vi "Simple Serial.vi"() -> ()   [LabVIEW 2021]
doc: "This example performs a serial port write and a serial port read. The parameters set for the serial port must match the parameters of the connected instrument or device. The VISA Configure Serial Port VI sets the configuration parameters. The front panel displays the controls used to configure the basic parameters, such as baud rate, data bits, and parity. The VI passes the VISA resource name to other VIs that perform operations on that VISA resource. The VISA Write function sends a command to the serial device and the VISA Read function returns data based on the command. The VISA Close function then closes the reference to the serial device. It is important to close the reference; otherwise, further communication through that port might not be possible."
uses:
  <vilib>/Instr/_visa.llb/VISA Open Access Mode.ctl
  <vilib>/Instr/_visa.llb/VISA Configure Serial Port (Instr).vi
panel:
  in  "Command":string="CAB-2558\n"
  out "bytes read":u32
  in  "delay before read (ms)":u32=500
  out "Response":string
  in  "VISA resource name":refnum<visa-resource-name>="COM1"
  # "Overview: Demonstrates the use of the VISA functions to send a single command to a serial instrument and read a response.\nRequirements: NI-VISA Driver\nInstructions:\n1. Ensure the resource specified by the VISA resource name is a valid serial device.\n2. Run the VI.\n3. If your instrument recognizes the \"*IDN?\" command, it should return a Response."
  # "Note: For an example of how to perform continuous serial communication in a loop, open the Continuous Serial Write and Read.vi in the same folder as this example."
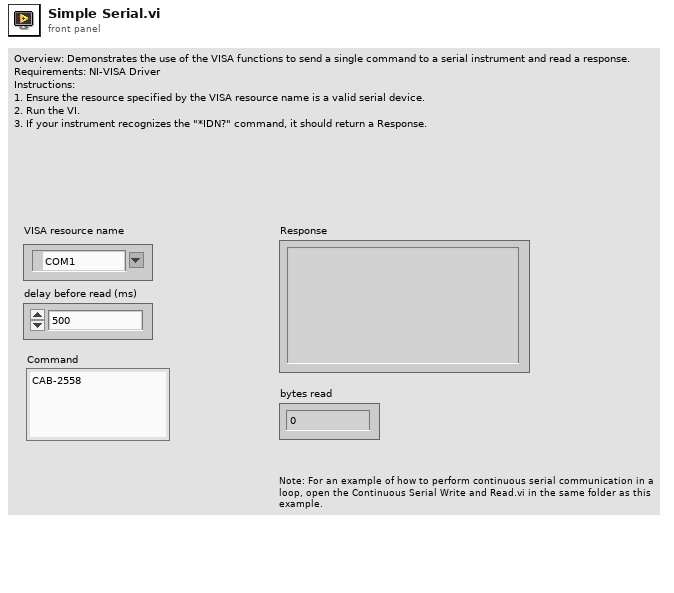
[diagram p1: front panel]
types:
  T1 = typedef "VISA Open Access Mode.ctl" = u32
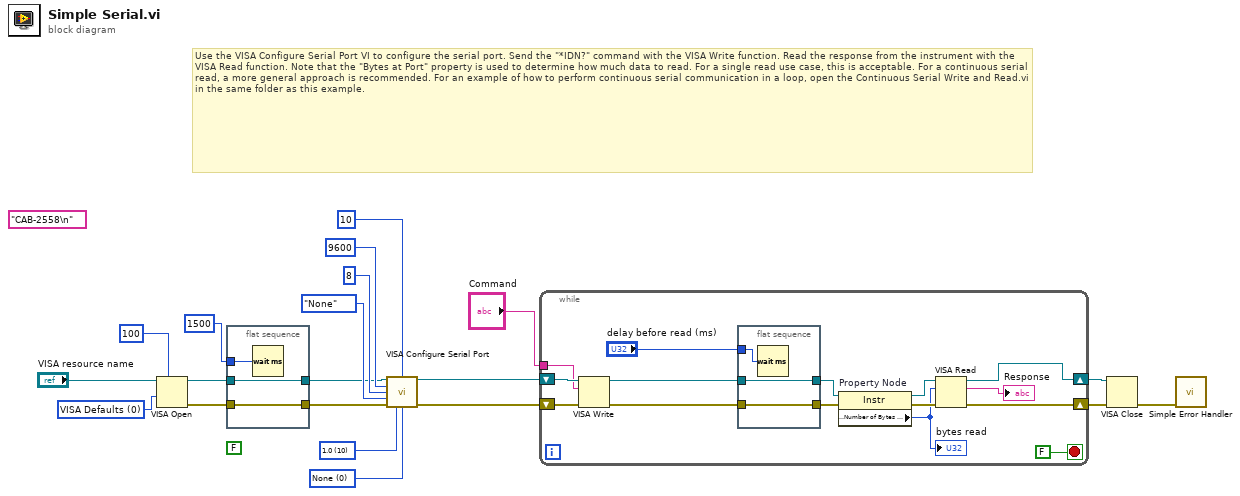
[diagram p0: block diagram]
diagram:
  (unwired) "CAB-2558\n" ("Command")
  (unwired) FALSE
  w11 = T1 0 items=["VISA Defaults"=0, "Exclusive Lock"=1, "Load Configured Settings"=4] ("Access Mode")
  w13 = u16 0 items=["None", "XON/XOFF", "RTS/CTS", "XON/XOFF & RTS/CTS", "DTR/DSR", "XON/XOFF & DTR/DSR"] ("flow control (0:none)")
  w14 = u16 10 items=["1.0"=10, "1.5"=15, "2.0"=20] ("stop bits (10: 1 bit)")
  # "Use the VISA Configure Serial Port VI to configure the serial port. Send the \"*IDN?\" command with the VISA Write function. Read the response from the instrument with the VISA Read function. Note that the \"Bytes at Port\" property is used to determine how much data to read. For a single read use case, this is acceptable. For a continuous serial read, a more general approach is recommended. For an example of how to perform continuous serial communication in a loop, open the Continuous Serial Write and Read.vi in the same folder as this example."
  n1 = VISA Open(timeout (0)=u32 100 ("VISA Open timeout (0)"), access mode=w11, VISA resource name="VISA resource name") -> (VISA resource name=w4:refnum<visa-resource-name>, error out=w2:errorcluster)  [unwired: 2 in]
  n2 = flat-sequence {
    tunnel: u32 1500 ("milliseconds to wait") -> [w23]
    tunnel: [w22] -> w5
    tunnel: w4 -> [w22]
    tunnel: [w21] -> w3
    tunnel: w2 -> [w21]
    frame #0 {
      n3 = Wait (ms)(milliseconds to wait=w23) -> ()  [unwired: 1 out]
    }
  }
  n4 = call-poly "VISA Configure Serial Port"("VISA resource name"=w5, "termination char\n(0xA = '\\n' = LF)"=u8 10 ("termination char\n(0xA = '\\n' = LF)"), "baud rate (9600)"=u32 9600, "data bits (8)"=u16 8, "parity (0:none)"=enum16{"None", "Odd", "Even", "Mark", "Space"}."None", "error in (no error)"=w3, "stop bits (10: 1 bit)"=w14, "flow control (0:none)"=w13) -> ("VISA resource name out"=w8:refnum<visa-resource-name>, "error out"=w9:errorcluster)  [unwired: 2 in, 4 out]
  n5 = while {
    tunnel: "Command" -> [w26]
    shift-right: [w38] -> w20
    shift-left: w9 -> [w32]
    shift-right: [w37] -> w19
    shift-left: w8 -> [w31]
    stop <- FALSE stop-if-true
    n6 = VISA Write(VISA resource name=w31, write buffer=w26, error in (no error)=w32) -> (VISA resource name out=w28:refnum<visa-resource-name>, error out=w30:errorcluster)  [unwired: 1 out]
    n7 = flat-sequence {
      tunnel: w30 -> [w40]
      tunnel: [w40] -> w29
      tunnel: w28 -> [w39]
      tunnel: [w39] -> w27
      tunnel: "delay before read (ms)" -> [w41]
      frame #0 {
        n8 = Wait (ms)(milliseconds to wait=w41) -> ()  [unwired: 1 out]
      }
    }
    n9 = property on="Property Node" class="Instr"(reference=w27, error in=w29) -> (reference out=w36:refnum<visa-resource-name>, error out=w35:errorcluster, "Serial Settings:Number of Bytes at Serial Port"=w34:u32)
    "bytes read" <- w34
    n10 = VISA Read(VISA resource name=w36, byte count=w34, error in (no error)=w35) -> (VISA resource name out=w37:refnum<visa-resource-name>, read buffer=→"Response":string, error out=w38:errorcluster)  [unwired: 1 out]
  }
  n11 = VISA Close(VISA resource name=w19, error in (no error)=w20) -> (error out=w18:errorcluster)
  n12 = call <vilib>:"Simple Error Handler.vi"("error in (no error)"=w18) -> ()  [unwired: 1 in, 8 out]
